vi "4.1 Arguments - Complex Data As Arguments.vi"() -> ()   [LabVIEW 2017]
uses:
  user.lib/_NEVSTOP/Communicable State Machine(CSM)/Communicable State Machine.lvlib
  user.lib/_NEVSTOP/Communicable State Machine(CSM)/_Shared/CSM Shared.lvlib
panel:
  out "Arg Token":string
  out "HEX String (0-9,A-F) 2":string="1400800000000002000D400300074E756D65726963001240400001FFFFFFFF0000054172726179000100010000000500000241000081790000002C000001640000002D00000000"
  out "HEX String (0-9,A-F)":string="1400800000000005000C40210673746174757300000B40030004636F64650000104030FFFFFFFF06736F757263650000104030FFFFFFFF06737472696E67000022405000040000000100020003136572726F7220696E20286E6F206572726F7229000100040100038BF000000033436865636B20596F757220496E7465726E65742053706565642077697468206F7572205370656564205465737420546F6F6C2000000033436865636B20596F757220496E7465726E65742053706565642077697468206F7572205370656564205465737420546F6F6C2000000000"
  out "Array 2":i32[](array[numeric])=[577, 33145, 44, 356, 45]
  in  "Array":i32[](array[numeric])=[577, 33145, 44, 356, 45]
  out "value":T1={"status"=TRUE, "code"=232432, "source"="Check Your Internet Speed with our Speed Test Tool ", "string"="Check Your Internet Speed with our Speed Test Tool "}
  in  "error in (no error)":T1={"status"=TRUE, "code"=232432, "source"="Check Your Internet Speed with our Speed Test Tool ", "string"="Check Your Internet Speed with our Speed Test Tool "}
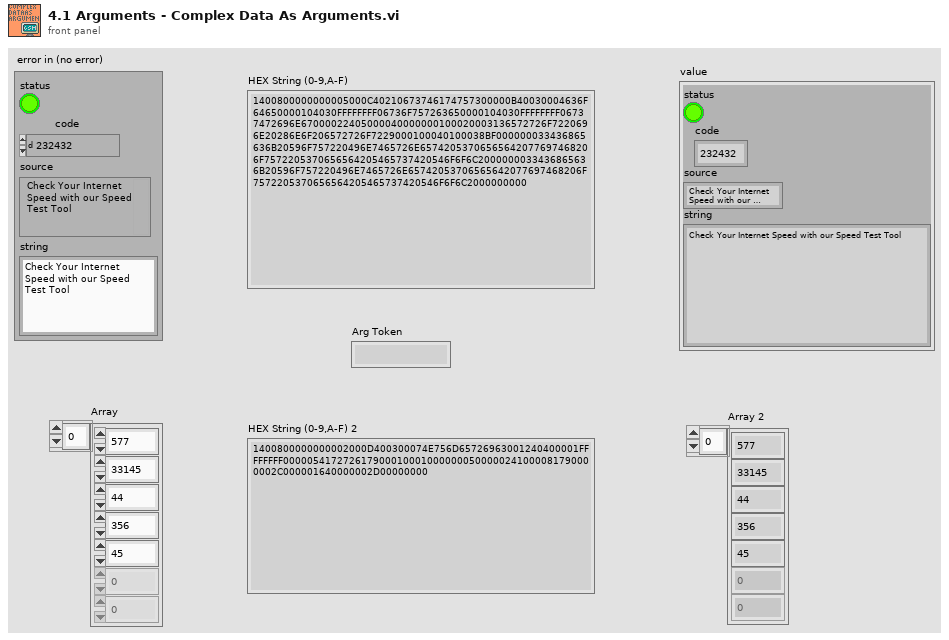
[diagram p1: front panel]
types:
  T1 = cluster{"status":bool, "code":i32, "source":string, "string":string}
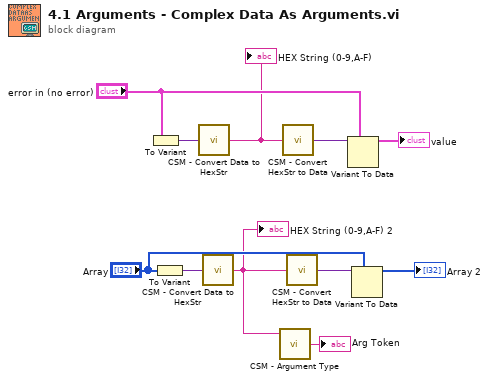
[diagram p0: block diagram]
diagram:
  n1 = To Variant(anything="error in (no error)") -> (Variant=w9:variant)
  n2 = To Variant(anything="Array") -> (Variant=w5:variant)
  n3 = call "CSM - Convert Data to HexStr.vi"("Variant"=w9) -> ("HEX String (0-9,A-F)"=w8:string)  [unwired: 8 in]
  "HEX String (0-9,A-F)" <- w8
  n4 = call "CSM - Convert Data to HexStr.vi"("Variant"=w5) -> ("HEX String (0-9,A-F)"=w2:string)  [unwired: 8 in]
  "HEX String (0-9,A-F) 2" <- w2
  n5 = call "CSM - Argument Type.vi"("Arguments"=w2) -> ("Argument Type"=→"Arg Token":string)  [unwired: 3 in, 1 out]
  n6 = call "CSM - Convert HexStr to Data.vi"("HEX String"=w8) -> ("Variant"=w7:variant)  [unwired: 7 in, 1 out]
  n7 = call "CSM - Convert HexStr to Data.vi"("HEX String"=w2) -> ("Variant"=w6:variant)  [unwired: 7 in, 1 out]
  n8 = Variant To Data(type="error in (no error)", Variant=w7) -> (data=→"value":T1)  [unwired: 1 in, 1 out]
  n9 = Variant To Data(type="Array", Variant=w6) -> (data=→"Array 2":i32[])  [unwired: 1 in, 1 out]
